vi "get connected terminals.vi"(7 "exclusions":refnum<vi>[](array[refnum]), 8 "error in":errorcluster, 11 "all terms":refnum<vi>[](array[refnum])) -> (0 "error out":errorcluster, 3 "linked terms":refnum<vi>[](array[refnum]))   [LabVIEW 2013, in "NISE Tools Scripting.lvlib"]
uses:
  NISE Tools Scripting.lvlib
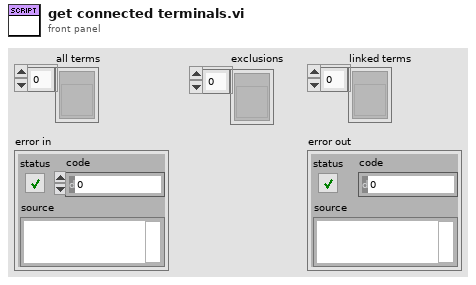
[diagram p1: front panel]
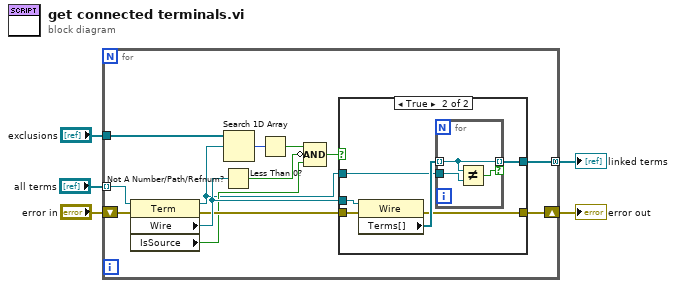
[diagram p0: block diagram]
diagram:
  n1 = for {
    tunnel: "all terms" -> [w18] mode=indexing
    tunnel: "exclusions" -> [w9]
    shift-right: [w13] -> w3
    shift-left: "error in" -> [w17]
    tunnel: [w11] -> w2 mode=concatenating
    n2 = property class="Term"(reference=w18, error in=w17) -> (reference out=w8:refnum<vi>, error out=w12:errorcluster, "Wire"=w14:refnum<vi>, "IsSource"=w10:bool)
    n3 = Not A Number/Path/Refnum?(number/path/refnum=w14) -> (NaN/Path/Refnum?=w16:bool)
    n4 = Search 1D Array(1D array=w9, element=w8) -> (index of element=w7:i32)  [unwired: 1 in]
    n5 = Less Than 0?(x=w7) -> (x < 0?=w6:bool)
    n6 = Compound Arithmetic op=AND(w6, invert w16, w10) -> (w15:bool)
    n7 = case shown="True" w15 {
      tunnel: w14 -> [_ w25]
      tunnel: [w19 w20] -> w13
      tunnel: w12 -> [w19 w24]
      tunnel: w8 -> [_ w22]
      tunnel: [_ w21] -> w11
      frame False {
      }
      frame True {
        n8 = property class="Wire"(reference=w25, error in=w24) -> (error out=w20:errorcluster, "Terms[]"=w23:refnum<vi>[])  [unwired: 1 out]
        n9 = for {
          tunnel: w23 -> [w27] mode=indexing
          tunnel: w22 -> [w28]
          tunnel: [w27] -> w21 mode=indexing if=w26
          n10 = Not Equal?(x=w27, y=w28) -> (x != y?=w26:bool)
        }
      }
    }
  }
  "error out" <- w3
  "linked terms" <- w2
